vi "read line from table.vi"(8 "error in":errorcluster, 10 "line number":i32, 11 "channels table":T2) -> (0 "error out":errorcluster, 1 "line":T1, 2 "empty tag?":bool, 3 "empty channel?":bool)   [LabVIEW 2014, in "alarms module editor node.lvclass"]
uses:
  alarms module editor node.lvclass
  table reference.ctl
  table line.ctl
  <vilib>/NI/Tag Bus Module Framework/channel/TBM channel.lvclass
  <vilib>/NI/Tag Bus/tag/tag descriptor.lvclass/tag descriptor.ctl
  <vilib>/NI/Tag Bus/tag/read tag name.vi
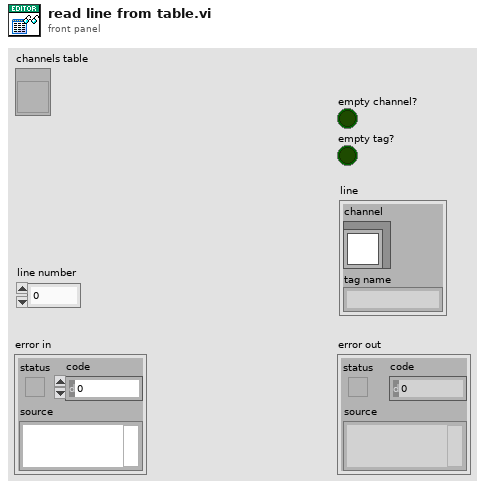
[diagram p1: front panel]
types:
  T1 = typedef "alarms module editor node.lvclass/table line.ctl" = cluster{"channel":refnum<class "TBM channel.lvclass">, "tag name":string}
  T2 = typedef "alarms module editor node.lvclass/table reference.ctl" = refnum<vi>
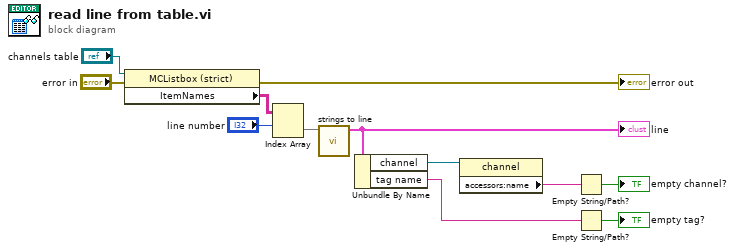
[diagram p0: block diagram]
diagram:
  n1 = property class="MCListbox (strict)"(reference="channels table", error in="error in") -> (error out=→"error out":errorcluster, "ItemNames"=w9:string[][])  [unwired: 1 out]
  n2 = Index Array(array=w9, index (row)="line number") -> (element=w7:string[])  [unwired: 1 in]
  n3 = call "strings to line.vi"("strings"=w7) -> ("line"=w6:T1)  [unwired: 10 in]
  "line" <- w6
  n4 = Unbundle By Name(w6) -> ("channel"=w5:refnum<class "TBM channel.lvclass">, "tag name"=w3:string)
  n5 = property class="channel"(reference=w5) -> ("accessors:name"=w4:string)  [unwired: 1 in, 2 out]
  n6 = Empty String/Path?(string/path=w4) -> (empty?=→"empty channel?":bool)
  n7 = Empty String/Path?(string/path=w3) -> (empty?=→"empty tag?":bool)
